vi "WPI_CameraSet Enum Sensor Property.vi"(7 "Strings":string[](array[string]), 8 "error in (no error)":errorcluster, 9 "Value":i32, 10 "Property Name":string, 11 "CameraDevRef":T1) -> (0 "error out":errorcluster, 3 "CameraDevRef Out":T1)   [LabVIEW 2017]
doc: "This software is licensed. Open the labview\\readme\\WPI Robotics Library Open Source License.txt file for more information."
uses:
  <vilib>/Rock Robotics/WPI/Camera/WPI_CameraDevRef.ctl
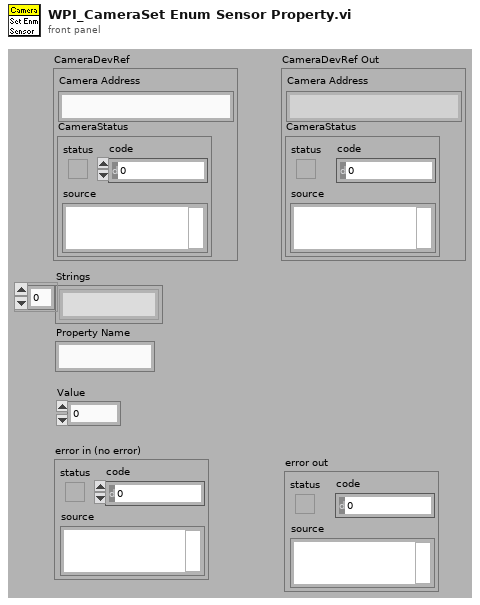
[diagram p1: front panel]
types:
  T1 = typedef "WPI_CameraDevRef.ctl" = cluster{"Camera Address":string, "CameraStatus":errorcluster}
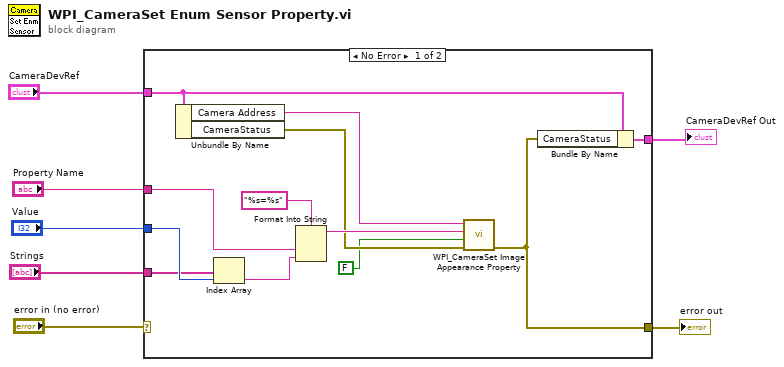
[diagram p0: block diagram]
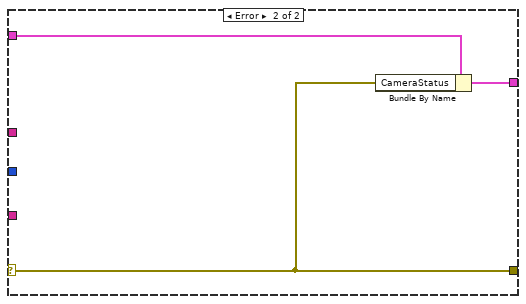
[diagram p2: hidden frame]
diagram:
  n1 = case shown="No Error" "error in (no error)" {
    selector: "error in (no error)" -> [_ w20]
    tunnel: [w12 w20] -> w7
    tunnel: [w19 w22] -> w6
    tunnel: "CameraDevRef" -> [w18 w21]
    tunnel: "Property Name" -> [w17 _]
    tunnel: "Value" -> [w15 _]
    tunnel: "Strings" -> [w13 _]
    frame No Error {
      n2 = Unbundle By Name(w18) -> ("Camera Address"=w8:string, "CameraStatus"=w10:errorcluster)
      n3 = Index Array(array=w13, index=w15) -> (element=w16:string)
      n4 = Format Into String(format string="%s=%s", w17, w16) -> (resulting string=w11:string)  [unwired: 2 in, 1 out]
      n5 = call <vilib>:"WPI_CameraSet Image Appearance Property.vi"("error in"=w10, "Appearance"=FALSE, "Prop String"=w11, "address"=w8) -> ("error out"=w12:errorcluster)  [unwired: 7 in]
      n6 = Bundle By Name(cluster=w18, "CameraStatus"=w12) -> (w19:T1)
    }
    frame Error {
      n7 = Bundle By Name(cluster=w21, "CameraStatus"=w20) -> (w22:T1)
    }
  }
  "error out" <- w7
  "CameraDevRef Out" <- w6
